vi "Check Goal Exist.vi"(8 "error in (no error)":errorcluster, 11 "Expense Summary in":refnum<class "Expense Summary.lvclass">) -> (0 "error out":errorcluster, 2 "Goal Exist?":bool, 3 "Expense Summary out":refnum<class "Expense Summary.lvclass">)   [LabVIEW 2018, in "Expense Summary.lvclass"]
uses:
  Expense Summary.lvclass
  Expense Summary.lvclass/Expense Summary.ctl
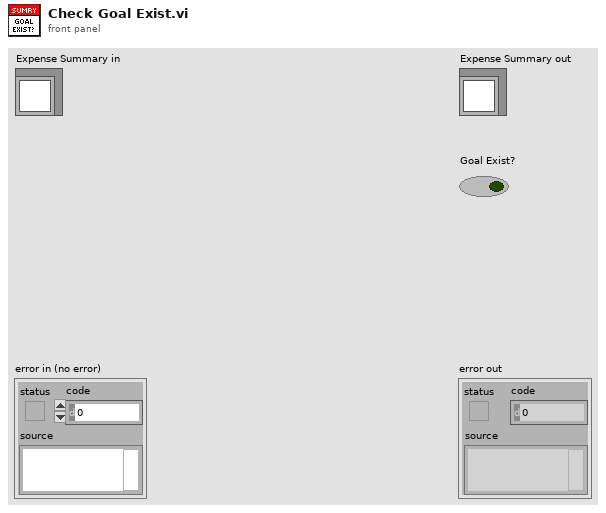
[diagram p1: front panel]
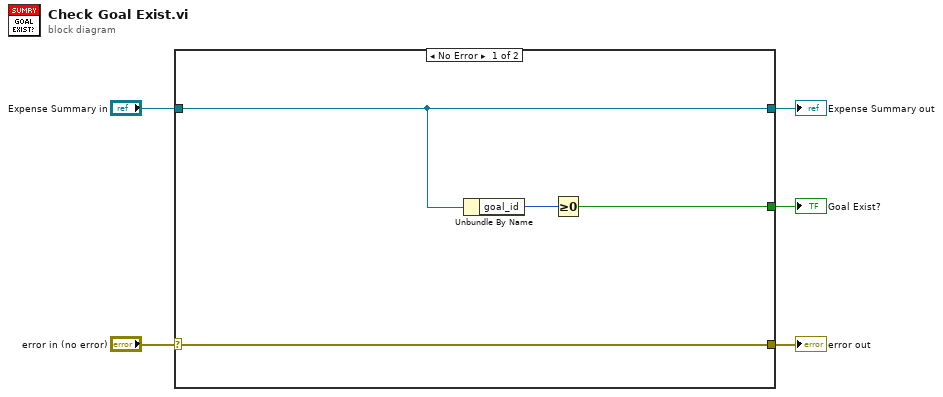
[diagram p0: block diagram]
diagram:
  n1 = case shown="No Error" "error in (no error)" {
    selector: "error in (no error)" -> [w9 w11]
    tunnel: [w9 w11] -> w4
    tunnel: [w8 w10] -> w2
    tunnel: "Expense Summary in" -> [w8 w10]
    tunnel: [w6 _] -> w1
    frame No Error {
      n2 = Unbundle By Name(w8) -> ("goal_id"=w7:i32)
      n3 = Greater Or Equal To 0?(x=w7) -> (x >= 0?=w6:bool)
    }
    frame Error {
    }
  }
  "error out" <- w4
  "Expense Summary out" <- w2
  "Goal Exist?" <- w1
